vi "GetType.vi"(8 "error in (no error)":errorcluster, 11 "Configure Sample Clock Output Enabled [SC] Msg in":refnum<class "Configure Sample Clock Output Enabled [SC] Msg.lvclass">) -> (0 "error out":errorcluster, 2 "Data Sample":variant, 3 "Configure Sample Clock Output Enabled [SC] Msg out":refnum<class "Configure Sample Clock Output Enabled [SC] Msg.lvclass">)   [LabVIEW 2014, in "CS++Fgen.lvlib" / "Configure Sample Clock Output Enabled [SC] Msg.lvclass"]
doc: "This VI delivers a sample of the data type format the message expects."
uses:
  Configure Sample Clock Output Enabled [SC] Msg.lvclass
  Configure Sample Clock Output Enabled [SC] Msg.lvclass/Configure Sample Clock Output Enabled [SC] Msg.ctl
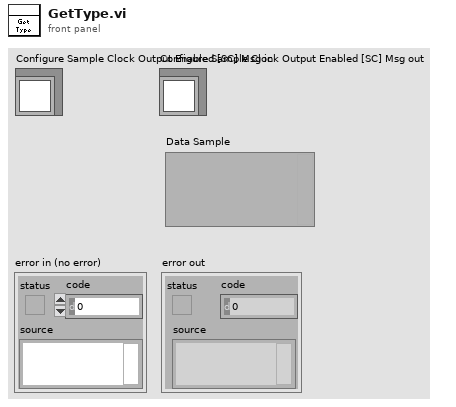
[diagram p1: front panel]
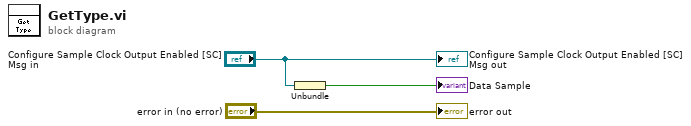
[diagram p0: block diagram]
diagram:
  n1 = Unbundle("Configure Sample Clock Output Enabled [SC] Msg in") -> (→"Data Sample":bool)
  "error out" <- "error in (no error)"
  "Configure Sample Clock Output Enabled [SC] Msg out" <- "Configure Sample Clock Output Enabled [SC] Msg in"
